vi "DCM DSI RT.vi"() -> ()   [LabVIEW 2016]
uses:
  <vilib>/addons/Software Calibration Management/xSCM/Controls/CalPoint - Data.ctl
  <vilib>/addons/Software Calibration Management/xSCM/Controls/CalPoint - Type.ctl
  <vilib>/addons/Software Calibration Management/xSCM/Controls/FaultPoint - Data.ctl
  <vilib>/addons/Software Calibration Management/xSCM/Controls/FaultPoint - Priority.ctl
  <vilib>/Platform/TimedLoop/XDataNode/timing_clust.ctl
  <vilib>/Platform/TimedLoop/XDataNode/nitl_modes.ctl
  <vilib>/Platform/TimedLoop/XDataNode/wakeup.ctl
  <vilib>/addons/Software Calibration Management/xSCM/CalPoint-Calibration File Path.vi
  <vilib>/addons/Software Calibration Management/xSCM/CalPoint-Load Calibration.vi
  <vilib>/addons/Software Calibration Management/xSCM/FaultPoint-Faults File Path.vi
  <vilib>/addons/Software Calibration Management/xSCM/FaultPoint-Load Faults.vi
  <vilib>/addons/Software Calibration Management/xSCM/CalPoint-Read Calibration.vi
  <vilib>/addons/Software Calibration Management/xSCM/SubVIs/Recompose Type.vi
  <vilib>/addons/Software Calibration Management/xSCM/FaultPoint-Read Faults.vi
  <vilib>/addons/Software Calibration Management/xSCM/FaultPoint-Set.vi
  <vilib>/addons/Software Calibration Management/xSCM/FaultPoint-Set Enabled.vi
  <vilib>/addons/Software Calibration Management/xSCM/FaultPoint-Set Acknowledged.vi
  <vilib>/addons/Software Calibration Management/xSCM/SubVIs/Match Element.vi
  <vilib>/addons/Software Calibration Management/xSCM/SubVIs/Variant Type Index.vi
  <vilib>/addons/Software Calibration Management/xSCM/SubVIs/Variant Element By Name.vi
  <vilib>/addons/Software Calibration Management/xSCM/SubVIs/Filter Calibration.vi
  <vilib>/addons/Software Calibration Management/xSCM/SubVIs/Remove Units Text.vi
  <vilib>/addons/Software Calibration Management/xSCM/SubVIs/A2L-Flatten Name.vi
  <vilib>/addons/Software Calibration Management/xSCM/CalPoint-Init.vi
  <vilib>/addons/Software Calibration Management/xSCM/CalPoint-Data.vi
  <vilib>/addons/Software Calibration Management/xSCM/SubVIs/Variant Data Index.vi
  <vilib>/addons/Software Calibration Management/xSCM/CalPoint-Set.vi
  <vilib>/addons/Software Calibration Management/xSCM/Set/Set Variant.vi
  <vilib>/addons/Software Calibration Management/xSCM/FaultPoint-Init.vi
  <vilib>/addons/Software Calibration Management/xSCM/FaultPoint-Data.vi
  <vilib>/addons/Software Calibration Management/xSCM/Servers/A2L-File/Launch.vi
  <vilib>/addons/Software Calibration Management/xSCM/Servers/ASAP3-MC-Ethernet/Launch.vi
  <vilib>/addons/Software Calibration Management/xSCM/Servers/Console-V4/Launch.vi
  <vilib>/addons/Software Calibration Management/xSCM/SCM Init.xnode
  <vilib>/addons/Software Calibration Management/xSCM/CalPoint.xnode
  <vilib>/Platform/TimedLoop/XDataNode/XDataNode.xnode
  <vilib>/Platform/TimedLoop/XDataNode/XDNodeRunTimeDep.lvlib
  RT/DSI-RT.lvlib
  <vilib>/Powertrain Controls/Device Drivers/DCM/Rev0/RT/DCM - RT.lvclass
  <vilib>/addons/Software Calibration Management/xSCM/ni_scm.dll
  Classes/DCM-DSI/DCM-DSI.lvclass
  <vilib>/addons/Software Calibration Management/xSCM/SCM-API.lvlib
  <vilib>/addons/Software Calibration Management/xSCM/Servers/A2L-File/SCM-A2L-File.lvclass
  <vilib>/addons/Software Calibration Management/xSCM/Servers/ASAP3-MC-Ethernet/SCM-ASAP3-MC-Ethernet.lvclass
  <vilib>/addons/Software Calibration Management/xSCM/Servers/Console-V4/SCM-Console-V4.lvclass
panel:
  out "System":i64(graph)
  in  "Stop":bool
  out "Monitor Loop Iteration":i32
  out "Command":i64(graph)
  out "SCMInitError":bool
  out "Init":errorcluster
  # "Powertrain Controls \nDCM\nDefault Software Image"
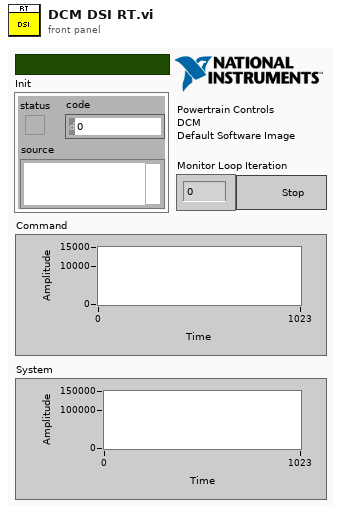
[diagram p1: front panel]
types:
  T1 = typedef "XDNodeRunTimeDep.lvlib/timing_clust.ctl" = cluster{"Expected End [f-1]":u64, "Actual End [f-1]":u64, "Finished Late? [f-1]":bool, "Expected End [i-1]":u64, "Actual End [i-1]":u64, "Finished Late? [i-1]":bool, "Expected Start [i]":u64, "Actual Start [i]":u64, "Expected Start [f]":u64, "Actual Start [f]":u64, "Source Name":string, "Structure Name":string, "Period":i64, "Deadline":i64, "Offset":i64, "Start":i64, "Priority":i32, "Timeout":i32, "Mode":T2, "Wakeup Reason":T3, "Error":errorcluster, "Source Type":string, "Secondary Source Type":string, "Global End Time":u64, "Global Start Time":u64, "Frame Duration":u64, "Iteration Duration":u64, "Assigned CPU":i32, "I/O Scan Engine Mode":u32}
  T2 = typedef "XDNodeRunTimeDep.lvlib/nitl_modes.ctl" = enum32{"No Change", "Process missed periods, maintain original phase", "Discard missed periods, maintain original phase", "Process missed periods, ignore original phase", "Discard missed periods, ignore original phase"}
  T3 = typedef "XDNodeRunTimeDep.lvlib/wakeup.ctl" = enum32{"Normal", "Aborted", "Asynchronous wakeup", "Timing source error", "Timed loop error", "Timeout"}
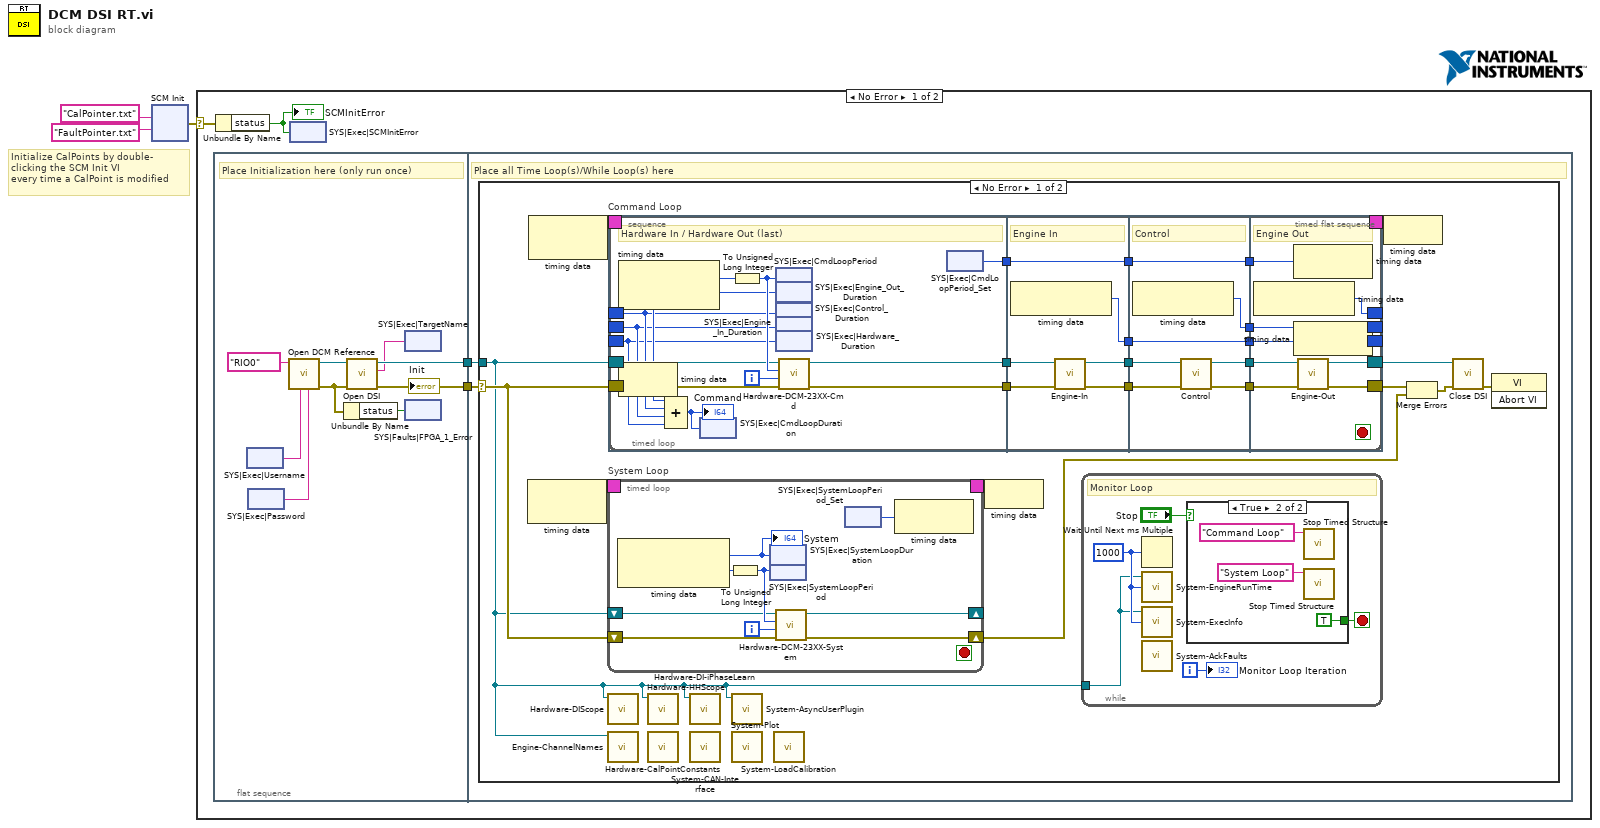
[diagram p0: block diagram]
diagram:
  # "Initialize CalPoints by double-\nclicking the SCM Init VI\nevery time a CalPoint is modified"
  n1 = xnode ("SCM Init")("Calibration"="CalPointer.txt" ("Calibration File"), "Faults"="FaultPointer.txt" ("Fault File")) -> ("Error"=w1:errorcluster)
  n2 = case shown="No Error" w1 {
    selector: w1 -> [w5 _]
    frame No Error {
      n3 = flat-sequence {
        tunnel: [w15] -> w7
        tunnel: [w16] -> w6
        tunnel: w7 -> [w52]
        tunnel: w6 -> [w51]
        frame #0 {
          # "Place Initialization here (only run once)"
          n4 = xnode "SYS|Exec|Username"() -> ("Value"=w10:string)
          n5 = xnode "SYS|Exec|Password"() -> ("Value"=w9:string)
          n6 = call <vilib>:"Open DCM Reference.vi"("Password"=w9, "User Name"=w10, "RIO"=tag "RIO0" ("resource name")) -> ("Error Out"=w12:errorcluster, "DCM Reference"=w13:refnum<class "DCM - RT.lvclass">)  [unwired: 7 in]
          n7 = Unbundle By Name(w12) -> ("status"=w14:bool)
          n8 = call "Open DSI.vi"("error in (no error)"=w12, "DCM"=w13) -> ("error out"=w15:errorcluster, "Target Name"=w11:string, "DSI Reference"=w16:refnum<class "DCM-DSI.lvclass">)  [unwired: 7 in]
          "Init" <- w15
          n9 = xnode "SYS|Exec|TargetName"("Value"=w11) -> ()
          n10 = xnode "SYS|Faults|FPGA_1_Error"("Value"=w14) -> ()
        }
        frame #1 {
          # "Place all Time Loop(s)/While Loop(s) here"
          n11 = case shown="No Error" w52 {
            selector: w52 -> [w63 _]
            tunnel: w51 -> [w55 _]
            frame No Error {
              n12 = node-c288 ("Input Node")() -> (w54:T1)  [unwired: 1 in]
              n13 = node-c288 ("Input Node")() -> (w61:T1)  [unwired: 1 in]
              n14 = timed-loop "System Loop" {
                timing: w54 -> [_]
                timing-out: [_] -> w53
                shift-right: [w65] -> w62
                shift-left: w63 -> [w72]
                shift-right: [w66] -> _
                shift-left: w55 -> [w69]
                i -> [w67]
                stop <- _ stop-if-true
                n15 = node-c288 ("Output Node")() -> (w68:i64, w70:i64)  [unwired: 1 in]
                "System" <- w68
                n16 = To Unsigned Long Integer(number=w70) -> (unsigned 32bit integer=w71:u32)
                n17 = xnode "SYS|Exec|SystemLoopDuration"("Value"=w68) -> ()
                n18 = xnode "SYS|Exec|SystemLoopPeriod"("Value"=w71) -> ()
                n19 = call "Hardware-DCM-23XX-System.vi"("error in (no error)"=w72, "LoopCount"=w67, "LoopPeriod [usec]"=w71, "DSI Reference"=w69) -> ("error out"=w65:errorcluster, "DSI Reference"=w66:refnum<class "DCM-DSI.lvclass">)  [unwired: 6 in]
                n20 = xnode "SYS|Exec|SystemLoopPeriod_Set"() -> ("Value"=w64:u32)
                n21 = node-c288 ("Input Node")(w64) -> ()  [unwired: 1 out]
              }
              n22 = call "Hardware-DIScope.vi"("DSI Reference"=w55) -> ()  [unwired: 11 in]
              n23 = call "Engine-ChannelNames.vi"("DSI Reference"=w55) -> ()  [unwired: 11 in]
              n24 = timed-loop "Command Loop" {
                timing: w61 -> [_]
                timing-out: [_] -> w60
                shift-right: [w114] -> _
                shift-left: _ -> [w113]
                shift-right: [w110] -> _
                shift-left: _ -> [w112]
                shift-right: [w111] -> _
                shift-left: _ -> [w109]
                shift-right: [w107] -> w59
                shift-left: w63 -> [w108]
                shift-right: [w106] -> w56
                shift-left: w55 -> [w105]
                i -> [w137]
                stop <- _ stop-if-true
                n25 = timed-sequence {
                  timing: _ -> [_]
                  timing-out: _ -> [_]
                  tunnel: [w131] -> w114
                  tunnel: w113 -> [w130]
                  tunnel: w112 -> [w126]
                  tunnel: [w125] -> w111
                  tunnel: [w123] -> w110
                  tunnel: w109 -> [w122]
                  tunnel: w108 -> [w118]
                  tunnel: [w117] -> w107
                  tunnel: [w116] -> w106
                  tunnel: w105 -> [w115]
                  n26 = timed-flat-sequence {
                    tunnel: [w145] -> w136
                    tunnel: w130 -> [w141]
                    tunnel: [w147] -> w127
                    tunnel: w126 -> [w142]
                    tunnel: w122 -> [w143]
                    tunnel: [w139] -> w121
                    tunnel: w118 -> [w148]
                    tunnel: w115 -> [w146]
                    tunnel: w136 -> [w190]
                    tunnel: [w189] -> w134
                    tunnel: [w191] -> w132
                    tunnel: [w187] -> w128
                    tunnel: w127 -> [w188]
                    tunnel: w121 -> [w186]
                    tunnel: [w186] -> w120
                    tunnel: [w198] -> w135
                    tunnel: w134 -> [w199]
                    tunnel: [w201] -> w133
                    tunnel: w132 -> [w201]
                    tunnel: [w196] -> w129
                    tunnel: w128 -> [w197]
                    tunnel: [w200] -> w124
                    tunnel: w120 -> [w195]
                    tunnel: [w195] -> w119
                    tunnel: w135 -> [w210]
                    tunnel: w133 -> [w212]
                    tunnel: [w212] -> w131
                    tunnel: w129 -> [w211]
                    tunnel: [w209] -> w125
                    tunnel: w124 -> [w208]
                    tunnel: [w208] -> w123
                    tunnel: w119 -> [w205]
                    tunnel: [w207] -> w117
                    tunnel: [w206] -> w116
                    frame #0 {
                      # "Hardware In / Hardware Out (last)"
                      n27 = node-c288 ("Output Node")() -> (w138:i64, w144:i64)  [unwired: 1 in]
                      n28 = Compound Arithmetic op=ADD(w144, w143, w142, w141) -> (w140:i64)
                      "Command" <- w140
                      n29 = xnode "SYS|Exec|CmdLoopDuration"("Value"=w140) -> ()
                      n30 = To Unsigned Long Integer(number=w138) -> (unsigned 32bit integer=w149:u32)
                      n31 = xnode "SYS|Exec|CmdLoopPeriod"("Value"=w149) -> ()
                      n32 = xnode "SYS|Exec|Engine_Out_Duration"("Value"=w144) -> ()
                      n33 = xnode "SYS|Exec|Control_Duration"("Value"=w143) -> ()
                      n34 = xnode "SYS|Exec|Engine_In_Duration"("Value"=w142) -> ()
                      n35 = xnode "SYS|Exec|Hardware_Duration"("Value"=w141) -> ()
                      n36 = call "Hardware-DCM-23XX-Cmd.vi"("error in (no error)"=w148, "LoopCount"=w137, "LoopPeriod [usec]"=w149, "DSI Reference"=w146) -> ("error out"=w147:errorcluster, "DSI Reference"=w145:refnum<class "DCM-DSI.lvclass">)  [unwired: 6 in]
                      n37 = xnode "SYS|Exec|CmdLoopPeriod_Set"() -> ("Value"=w139:u32)
                    }
                    frame #1 {
                      # "Engine In"
                      n38 = node-c288 ("Output Node")() -> (w191:i64)  [unwired: 1 in]
                      n39 = call "Engine-In.vi"("error in (no error)"=w188, "DSI Reference"=w190) -> ("error out"=w187:errorcluster, "DSI Reference"=w189:refnum<class "DCM-DSI.lvclass">)  [unwired: 8 in]
                    }
                    frame #2 {
                      # "Control"
                      n40 = node-c288 ("Output Node")() -> (w200:i64)  [unwired: 1 in]
                      n41 = call "Control.vi"("error in (no error)"=w197, "DSI Reference"=w199) -> ("error out"=w196:errorcluster, "DSI Reference"=w198:refnum<class "DCM-DSI.lvclass">)  [unwired: 8 in]
                    }
                    frame #3 {
                      # "Engine Out"
                      n42 = node-c288 ("Output Node")() -> (w209:i64)  [unwired: 1 in]
                      n43 = node-c288 ("Input Node")(w205) -> ()  [unwired: 1 out]
                      n44 = call "Engine-Out.vi"("error in (no error)"=w211, "DSI Reference"=w210) -> ("error out"=w207:errorcluster, "DSI Reference"=w206:refnum<class "DCM-DSI.lvclass">)  [unwired: 8 in]
                    }
                  }
                }
                n45 = node-c288 ("Output Node")() -> ()  [unwired: 1 in, 1 out]
                n46 = node-c288 ("Input Node")() -> ()  [unwired: 1 in, 1 out]
              }
              n47 = call "Hardware-HHScope.vi"("DSI Reference"=w55) -> ()  [unwired: 11 in]
              n48 = call "Hardware-CalPointConstants.vi"() -> ()  [unwired: 12 in]
              n49 = call "Hardware-DI-iPhaseLearn.vi"("DSI Reference"=w55) -> ()  [unwired: 11 in]
              n50 = call "System-CAN-Interface.vi"() -> ()  [unwired: 12 in]
              n51 = call "System-AsyncUserPlugin.vi"("DSI Reference"=w55) -> ()  [unwired: 11 in]
              n52 = call "System-Plot.vi"() -> ()  [unwired: 12 in]
              n53 = call "System-LoadCalibration.vi"() -> ()  [unwired: 12 in]
              n54 = node-c288 ("Output Node")(w53) -> ()
              n55 = while "Slow Speed Loop" {
                tunnel: w55 -> [w98]
                i -> [w101]
                stop <- w100 stop-if-true
                w99 = u32 1000 ("millisecond multiple")
                # "Monitor Loop"
                n56 = Wait Until Next ms Multiple(millisecond multiple=w99) -> ()  [unwired: 1 out]
                n57 = call "System-EngineRunTime.vi"("Loop Period [ms]"=w99, "DSI Reference"=w98) -> ()  [unwired: 1 in]
                n58 = call "System-ExecInfo.vi"("Loop Period [ms]"=w99, "DSI Reference"=w98) -> ()  [unwired: 1 in]
                n59 = call "System-AckFaults.vi"() -> ()  [unwired: 12 in]
                n60 = case shown="True" "Stop" {
                  tunnel: [_ TRUE] -> w100
                  frame False {
                  }
                  frame True {
                    n61 = call <vilib>:"Stop Timed Structure.vi"("name"="Command Loop") -> ()  [unwired: 10 in, 1 out]
                    n62 = call <vilib>:"Stop Timed Structure.vi"("name"="System Loop") -> ()  [unwired: 10 in, 1 out]
                  }
                }
                "Monitor Loop Iteration" <- w101
              }
              n63 = node-c288 ("Output Node")(w60) -> ()
              n64 = Merge Errors(w59, w62) -> (w58:errorcluster)
              n65 = call "Close DSI.vi"("error in"=w58, "DSI Reference"=w56) -> ("error out"=w57:errorcluster)  [unwired: 9 in]
              n66 = invoke class="VI" method="Abort VI"(error in=w57) -> ()  [unwired: 2 in, 3 out]
            }
            frame Error {
            }
          }
        }
      }
      n67 = Unbundle By Name(w5) -> ("status"=w4:bool)
      "SCMInitError" <- w4
      n68 = xnode "SYS|Exec|SCMInitError"("Value"=w4) -> ()
    }
    frame Error {
    }
  }
